vi "FeedbackDecode_GenWfBuff.vi"(1 "ClearWfs":bool, 2 "WfCnt":i32, 3 "Wf":sgl[](array[numeric])) -> (0 "WfBuff":dbl[][](array[numeric]))   [LabVIEW 2020]
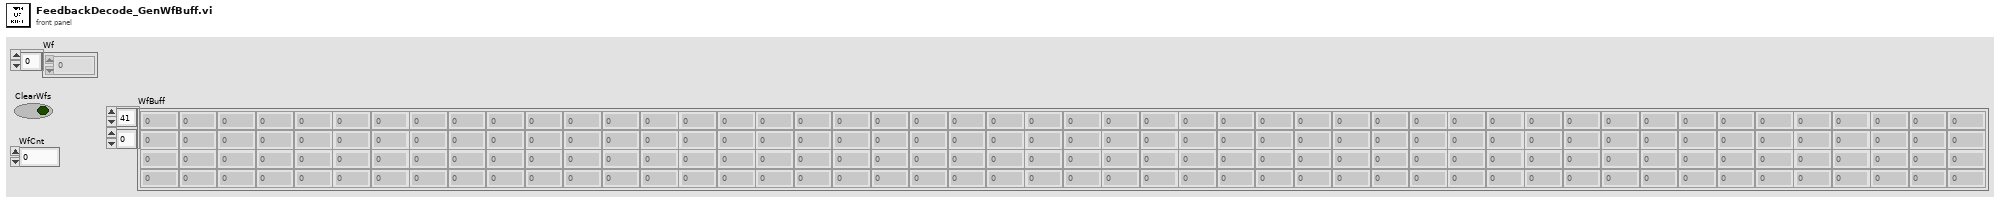
[diagram p1: front panel]
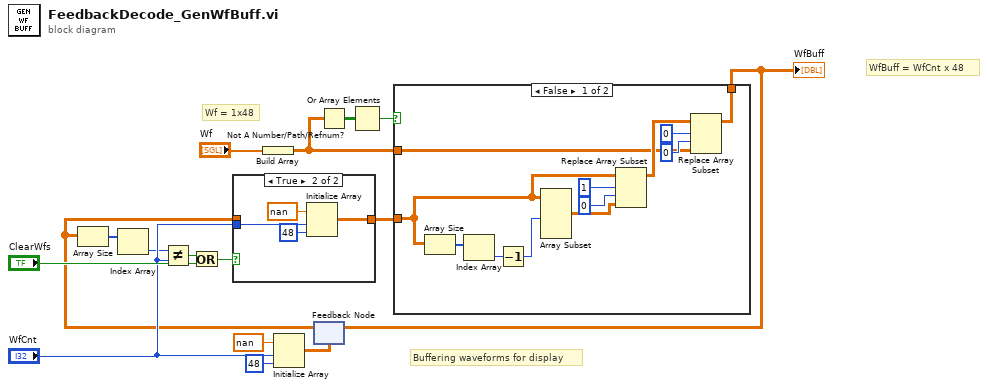
[diagram p0: block diagram]
diagram:
  # "WfBuff = WfCnt x 48"
  # "Wf = 1x48"
  # "Buffering waveforms for display"
  n1 = Build Array("Wf") -> (w16:sgl[][])
  n2 = Initialize Array(nan ("element"), "WfCnt", 48 ("dimension size")) -> (w1:dbl[][])
  n3 = feedback #1(w1) -> (w4:dbl[][])
  n4 = Array Size(array=w4) -> (size(s)=w5:i32[])
  n5 = Index Array(array=w5) -> (element=w6:i32)  [unwired: 1 in]
  n6 = Not Equal?(x=w6, y="WfCnt") -> (x != y?=w9:bool)
  n7 = Or(x=w9, y="ClearWfs") -> (x .or. y?=w11:bool)
  n8 = case shown="True" w11 {
    tunnel: w4 -> [w17 _]
    tunnel: [w17 w19] -> w3
    tunnel: "WfCnt" -> [_ w18]
    frame False {
    }
    frame True {
      n9 = Initialize Array(nan ("element"), w18, 48 ("dimension size")) -> (w19:dbl[][])
    }
  }
  n10 = Not A Number/Path/Refnum?(number/path/refnum=w16) -> (NaN/Path/Refnum?=w14:bool[][])
  n11 = Or Array Elements(Boolean array=w14) -> (logical OR=w13:bool)
  n12 = case shown="False" w13 {
    tunnel: w3 -> [w30 w34]
    tunnel: w16 -> [w22 _]
    tunnel: [w23 w34] -> w8
    frame False {
      n13 = Array Size(array=w30) -> (size(s)=w33:i32[])
      n14 = Index Array(array=w33) -> (element=w32:i32)  [unwired: 1 in]
      n15 = Decrement(x=w32) -> (x-1=w31:i32)
      n16 = Array Subset(array=w30, length (row)=w31) -> (w29:dbl[][])  [unwired: 3 in]
      n17 = Replace Array Subset(array=w30, new element=w29, index (row)=1, index (col)=0 ("disabled index (col)")) -> (w26:dbl[][])
      n18 = Replace Array Subset(array=w26, new element=w22, index (row)=0, index (col)=0 ("disabled index (col)")) -> (w23:dbl[][])
    }
    frame True {
    }
  }
  "WfBuff" <- w8
  n19 = feedback-in #1(w8) -> ()
